vi "FTW-Math-MovingAverage.vi"(2 "Reset?":bool, 5 "New Value":dbl, 9 "Window Size":i32=100) -> (6 "Average Value":dbl, 8 "Average dV/dt":dbl, 10 "Items in Window":i32)   [LabVIEW 2015]
panel:
  # "Inputs"
  # "Outputs"
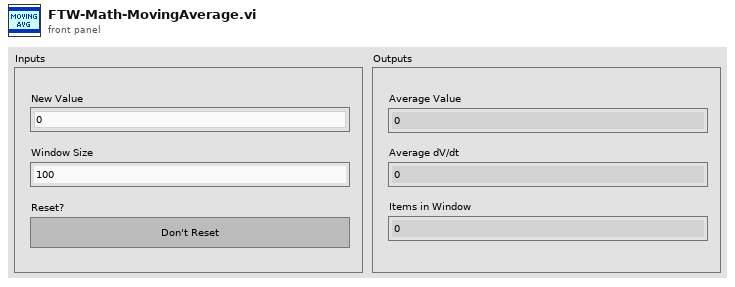
[diagram p1: front panel]
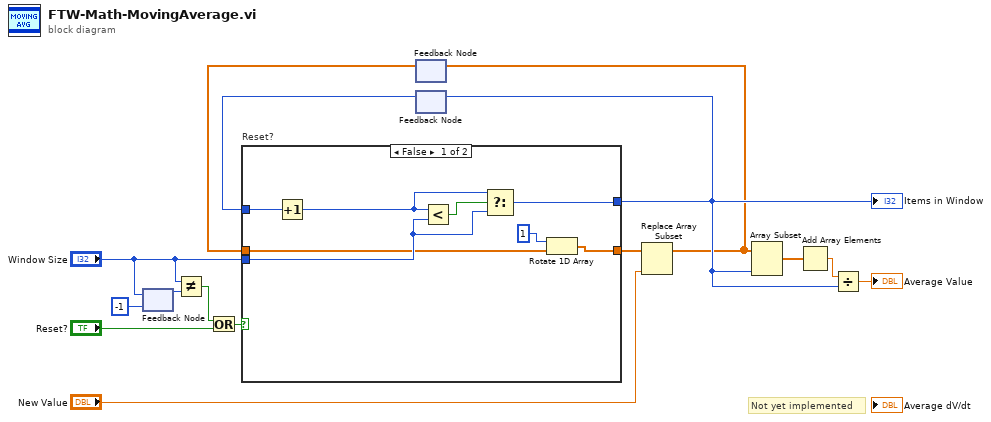
[diagram p0: block diagram]
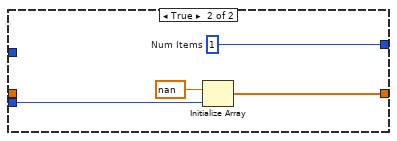
[diagram p2: hidden frame]
diagram:
  # "Not yet implemented"
  n1 = feedback #1(-1 ("Window Size")) -> (w4:i32)
  n2 = feedback-in #1("Window Size") -> ()
  n3 = Not Equal?(x="Window Size", y=w4) -> (x != y?=w2:bool)
  n4 = Or(x=w2, y="Reset?") -> (x .or. y?=w14:bool)
  n5 = feedback #2() -> (w13:dbl[])  [unwired: 1 in]
  n6 = feedback #3() -> (w12:i32)  [unwired: 1 in]
  n7 = case "Reset?" shown="False" w14 {
    tunnel: "Window Size" -> [w21 w27]
    tunnel: w13 -> [w19 _]
    tunnel: [w18 w25] -> w6
    tunnel: [w23 w24] -> w9
    tunnel: w12 -> [w22 _]
    frame False {
      n8 = Increment(x=w22) -> (x+1=w16:i32)
      n9 = Less?(x=w16, y=w21) -> (x < y?=w20:bool)
      n10 = Select(t=w16, s=w20, f=w21) -> (s? t:f=w23:i32)
      n11 = Rotate 1D Array(1:w19, 2:1 ("n")) -> (0:w18:dbl[])
    }
    frame True {
      w24 = 1  # Num Items
      n12 = Initialize Array(nan ("element"), w27) -> (w25:dbl[])
    }
  }
  "Items in Window" <- w9
  n13 = feedback-in #3(w9) -> ()
  n14 = Replace Array Subset(array=w6, new element="New Value") -> (w7:dbl[])  [unwired: 1 in]
  n15 = feedback-in #2(w7) -> ()
  n16 = Array Subset(array=w7, length=w9) -> (w11:dbl[])  [unwired: 1 in]
  n17 = Add Array Elements(numeric array=w11) -> (sum=w10:dbl)
  n18 = Divide(x=w10, y=w9) -> (x/y=→"Average Value":dbl)
